vi "随机数-for-延时.vi"() -> ()   [LabVIEW 2012]
panel:
  out "数值":dbl
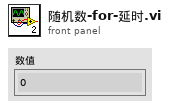
[diagram p1: front panel]
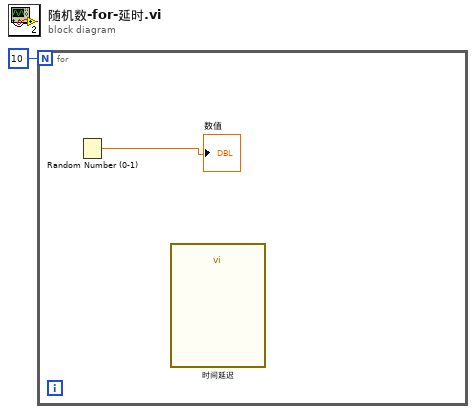
[diagram p0: block diagram]
diagram:
  n1 = for {
    N: 10 -> [_]
    n2 = Random Number (0-1)() -> (number: 0 to 1=→"数值":dbl)
    n3 = call "时间延迟"() -> ()  [unwired: 11 in, 1 out]
  }
